vi "Instrument Manager Loop.vi"(8 "System Control":refnum<queue>, 11 "Instrument Manager":refnum<queue>) -> (0 "error out":errorcluster)   [LabVIEW 2020, in "Mock Temperature Controller.lvlib" / "Instrument Manager.lvlib"]
uses:
  Instrument Manager/Instrument Manager.lvlib
  support/Message Queue/Message Cluster.ctl
  Instrument Manager/Instrument State.ctl
  <vilib>/Utility/error.llb/Error Cluster From Error Code.vi
  <vilib>/ErrorRing/Error Ring.xnode
  support/Message Queue/Message Queue.lvlib
  Mock Temperature Controller.lvlib
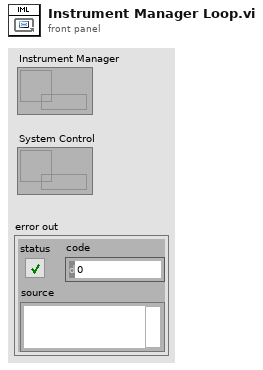
[diagram p1: front panel]
types:
  T1 = typedef "Mock Temperature Controller.lvlib/Instrument Manager.lvlib/Instrument State.ctl" = cluster{"VISA Resource":refnum<visa-resource-name>, "Setpoint":dbl, "Running":bool, "Running Since":timestamp, "Data Point":cluster{"Time Stamp":timestamp, "Value":dbl}, "Current Temperature":dbl, "Sampling Rate (sec/sample)":dbl}
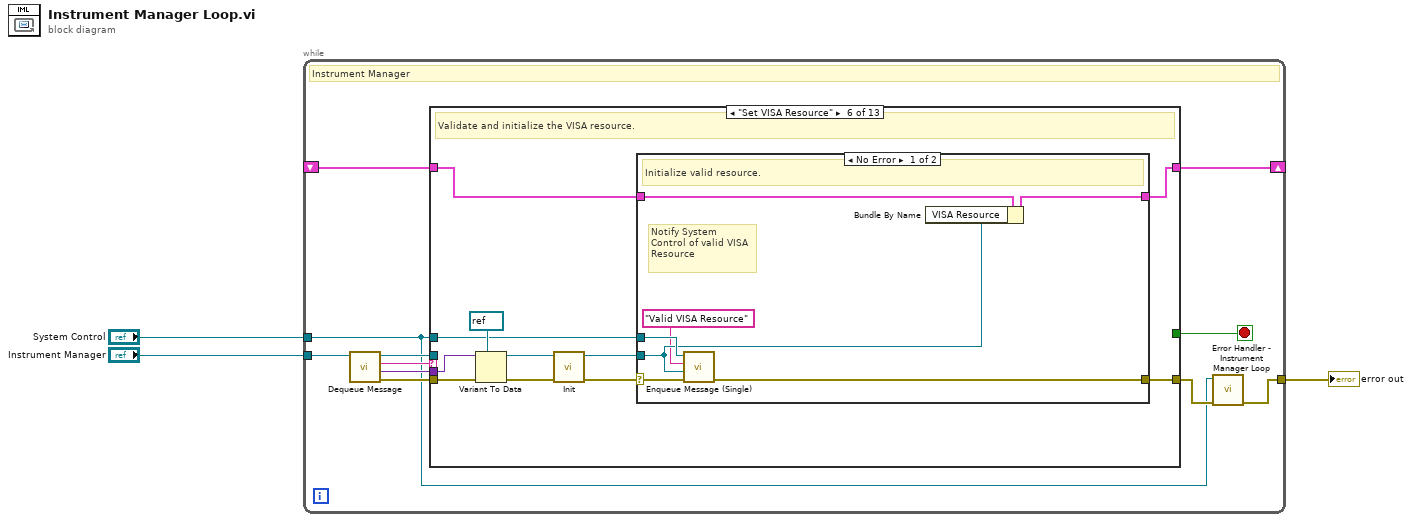
[diagram p0: block diagram]
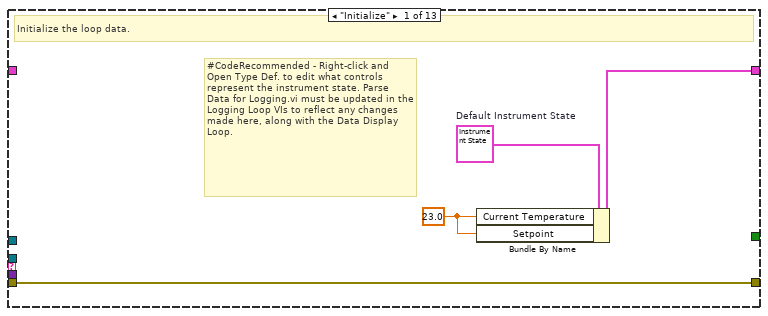
[diagram p2: hidden frame]
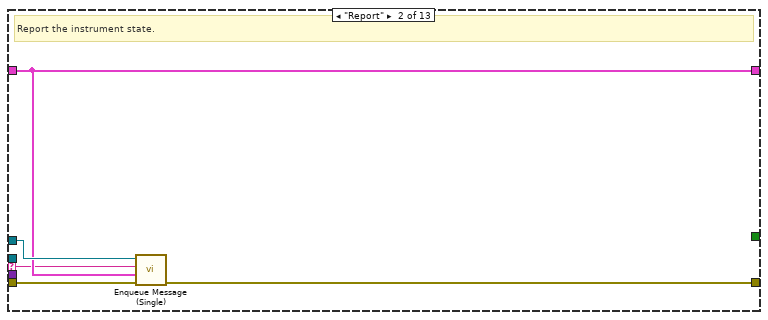
[diagram p3: hidden frame]
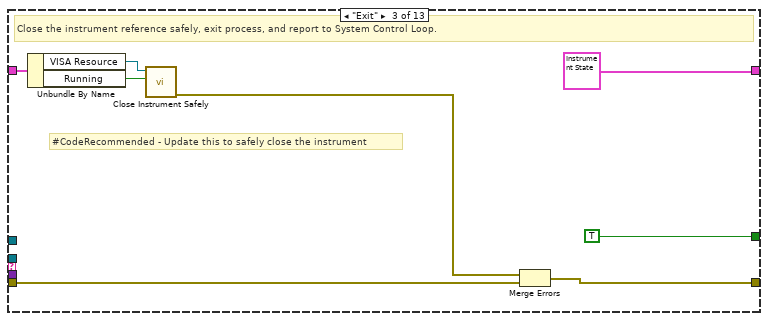
[diagram p4: hidden frame]
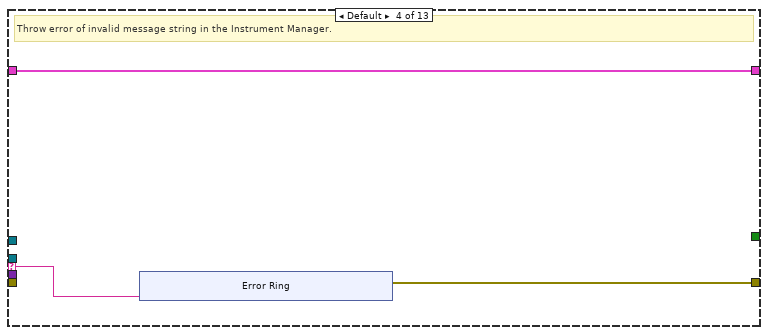
[diagram p5: hidden frame]
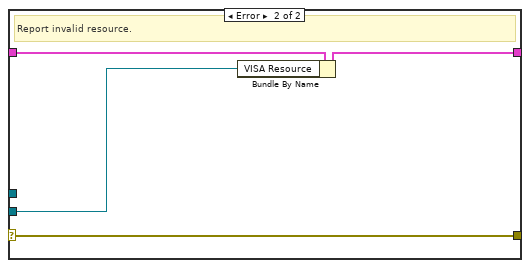
[diagram p7: hidden frame]
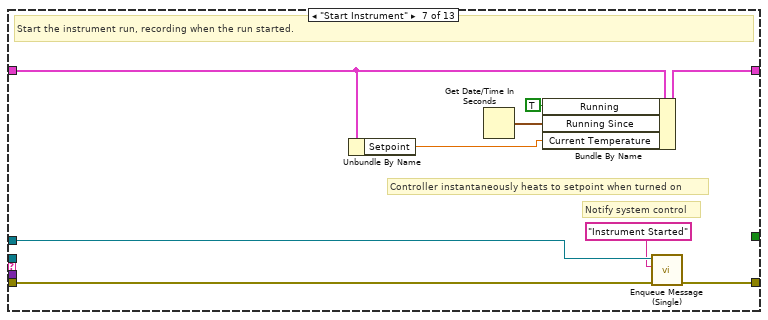
[diagram p8: hidden frame]
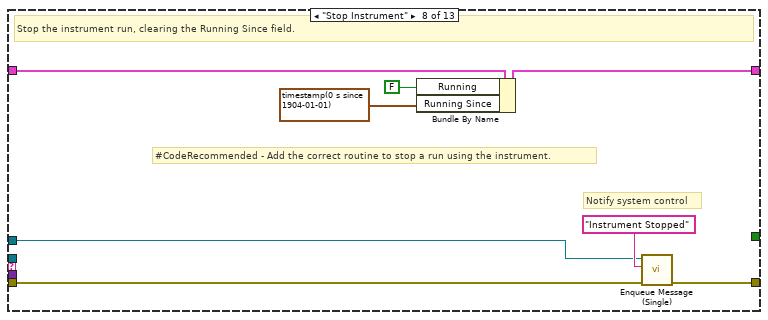
[diagram p9: hidden frame]
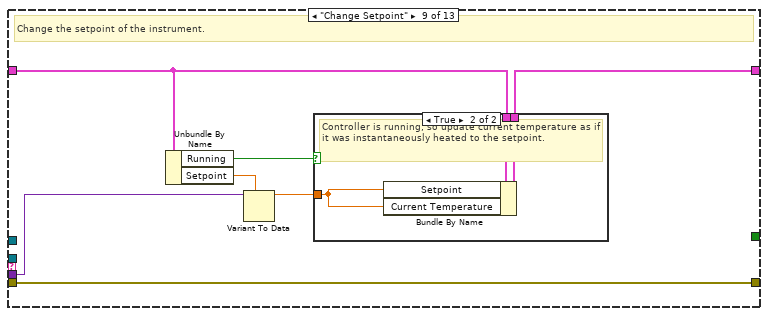
[diagram p10: hidden frame]
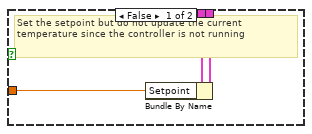
[diagram p11: hidden frame]
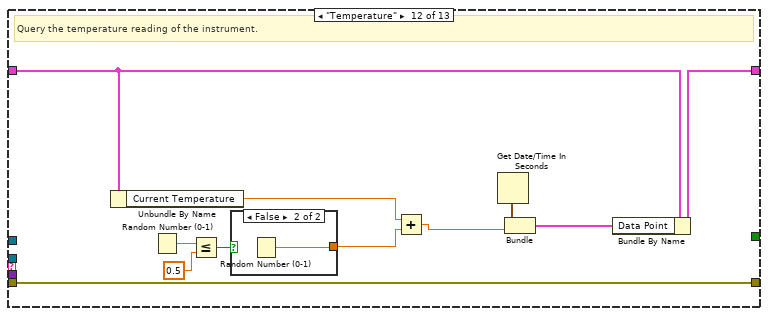
[diagram p14: hidden frame]
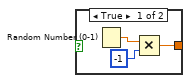
[diagram p15: hidden frame]
diagram:
  n1 = while {
    tunnel: "Instrument Manager" -> [w14]
    tunnel: "System Control" -> [w5]
    tunnel: [w8] -> w1
    shift-right: [w7] -> _
    shift-left: _ -> [w4]
    stop <- w6 stop-if-true
    # "Instrument Manager"
    n2 = call "Dequeue Message.vi"("Message Queue"=w14) -> ("error out"=w10:errorcluster, "Message Data"=w11:variant, "Message"=w13:string, "dup Message Queue"=w12:refnum<queue>)  [unwired: 7 in]
    n3 = case shown="\"Set VISA Resource\"" w13 {
      selector: w13 -> [_ w19 _ w33 _ _ _ _ _ _ _ _ _]
      tunnel: w12 -> [_ _ _ _ _ _ _ _ _ _ _ _ _]
      tunnel: w5 -> [_ w22 _ _ _ w44 w73 w80 _ _ _ _ _]
      tunnel: w11 -> [_ _ _ _ _ w51 _ _ w88 _ _ _ _]
      tunnel: w10 -> [w17 w23 w26 _ w42 w50 w68 w76 w85 w97 w99 w107 w116]
      tunnel: [w17 w21 w25 w32 w42 w54 w74 w82 w85 w97 w99 w107 w116] -> w9
      tunnel: w4 -> [_ w20 w31 w34 w43 w53 w67 w75 w87 w96 w98 w106 w115]
      tunnel: [w16 w20 T1 {"VISA Resource"="", "Setpoint"=0.0, "Running"=FALSE, "Running Since"=timestamp(0 s since 1904-01-01), "Data Point"={"Time Stamp"=timestamp(0 s since 1904-01-01), "Value"=0.0}, "Current Temperature"=0.0, "Sampling Rate (sec/sample)"=0.0} w34 w43 w52 w71 w79 w89 w96 w98 w110 w115] -> w7
      tunnel: [_ _ TRUE _ _ _ _ _ _ _ _ _ _] -> w6
      frame "Initialize" {
        w15 = 23.0 ("Current Temperature")
        w18 = T1 {"VISA Resource"="", "Setpoint"=0.0, "Running"=FALSE, "Running Since"=timestamp(0 s since 1904-01-01), "Data Point"={"Time Stamp"=timestamp(0 s since 1904-01-01), "Value"=0.0}, "Current Temperature"=0.0, "Sampling Rate (sec/sample)"=0.0}  # Default Instrument State
        # "#CodeRecommended - Right-click and Open Type Def. to edit what controls represent the instrument state. Parse Data for Logging.vi must be updated in the Logging Loop VIs to reflect any changes made here, along with the Data Display Loop."
        # "Initialize the loop data."
        n4 = Bundle By Name(cluster=w18, "Current Temperature"=w15, "Setpoint"=w15) -> (w16:T1)
      }
      frame "Report" {
        # "Report the instrument state."
        n5 = call "Enqueue Message (Single).vi"("error in (no error)"=w23, "Message Data"=w20, "Message"=w19, "Message Queue"=w22) -> ("error out"=w21:errorcluster)  [unwired: 6 in, 1 out]
      }
      frame "Exit" {
        # "#CodeRecommended - Update this to safely close the instrument"
        # "Close the instrument reference safely, exit process, and report to System Control Loop."
        n6 = Unbundle By Name(w31) -> ("VISA Resource"=w29:refnum<visa-resource-name>, "Running"=w30:bool)
        n7 = call "Close Instrument Safely.vi"("Running (F)"=w30, "VISA Refnum in"=w29) -> ("error out"=w24:errorcluster)  [unwired: 9 in]
        n8 = Merge Errors(w24, w26) -> (w25:errorcluster)
      }
      frame Default {
        # "Throw error of invalid message string in the Instrument Manager."
        n9 = xnode "Error Ring"("parameter 0"=w33) -> ("error out"=w32:errorcluster)
      }
      frame "--- Copy This Frame ---" {
        # "Copy this frame and add responses to instrument specific messages."
      }
      frame "Set VISA Resource" {
        # "Validate and initialize the VISA resource."
        n10 = Variant To Data(error in=w50, type=refnum<visa-resource-name> refnum, Variant=w51) -> (data=w48:refnum<visa-resource-name>, error out=w49:errorcluster)
        n11 = call "Init.vi"("error in (no error)"=w49, "VISA resource name"=w48) -> ("error out"=w45:errorcluster, "VISA resource out"=w46:refnum<visa-resource-name>)  [unwired: 8 in]
        n12 = case shown="No Error" w45 {
          selector: w45 -> [w60 w62]
          tunnel: w46 -> [w57 w63]
          tunnel: [w59 w62] -> w54
          tunnel: w53 -> [w61 w65]
          tunnel: [w55 w64] -> w52
          tunnel: w44 -> [w58 _]
          frame No Error {
            # "Notify System Control of valid VISA Resource"
            # "Initialize valid resource."
            n13 = call "Enqueue Message (Single).vi"("error in (no error)"=w60, "Message Data"=w57, "Message"="Valid VISA Resource", "Message Queue"=w58) -> ("error out"=w59:errorcluster)  [unwired: 6 in, 1 out]
            n14 = Bundle By Name(cluster=w61, "VISA Resource"=w57) -> (w55:T1)
          }
          frame Error {
            # "Report invalid resource."
            n15 = Bundle By Name(cluster=w65, "VISA Resource"=w63) -> (w64:T1)
          }
        }
      }
      frame "Start Instrument" {
        # "Controller instantaneously heats to setpoint when turned on"
        # "Notify system control"
        # "Start the instrument run, recording when the run started."
        n16 = Unbundle By Name(w67) -> ("Setpoint"=w66:dbl)
        n17 = Get Date/Time In Seconds() -> (seconds since 1Jan1904=w69:timestamp)
        n18 = Bundle By Name(cluster=w67, "Running"=TRUE, "Running Since"=w69, "Current Temperature"=w66) -> (w71:T1)
        n19 = call "Enqueue Message (Single).vi"("error in (no error)"=w68, "Message"="Instrument Started", "Message Queue"=w73) -> ("error out"=w74:errorcluster)  [unwired: 7 in, 1 out]
      }
      frame "Stop Instrument" {
        # "Notify system control"
        # "#CodeRecommended - Add the correct routine to stop a run using the instrument."
        # "Stop the instrument run, clearing the Running Since field."
        n20 = Bundle By Name(cluster=w75, "Running"=FALSE, "Running Since"=timestamp(0 s since 1904-01-01)) -> (w79:T1)
        n21 = call "Enqueue Message (Single).vi"("error in (no error)"=w76, "Message"="Instrument Stopped", "Message Queue"=w80) -> ("error out"=w82:errorcluster)  [unwired: 7 in, 1 out]
      }
      frame "Change Setpoint" {
        # "Change the setpoint of the instrument."
        n22 = Unbundle By Name(w87) -> ("Running"=w83:bool, "Setpoint"=w86:dbl)
        n23 = Variant To Data(type=w86, Variant=w88) -> (data=w84:dbl)  [unwired: 1 in, 1 out]
        n24 = case shown="True" w83 {
          tunnel: [w92 w94] -> w89
          tunnel: w87 -> [w91 w95]
          tunnel: w84 -> [w90 w93]
          frame False {
            # "Set the setpoint but do not update the current temperature since the controller is not running"
            n25 = Bundle By Name(cluster=w91, "Setpoint"=w90) -> (w92:T1)
          }
          frame True {
            # "Controller is running, so update current temperature as if it was instantaneously heated to the setpoint."
            n26 = Bundle By Name(cluster=w95, "Setpoint"=w93, "Current Temperature"=w93) -> (w94:T1)
          }
        }
      }
      frame "--- Copy for Get State Messages ---" {
        # "#CodeNeeded - Use the Bundle by Name function to bundle the new state value into the Instrument State cluster."
        # "#CodeNeeded - Add instrument driver call to query the instrument state requested"
        # "Duplicate this case for messages cases that will query the instrument state."
      }
      frame "Run State" {
        # "In a mock system this doesn't have to do anything"
        # "Query the run state of the instrument."
      }
      frame "Temperature" {
        # "Query the temperature reading of the instrument."
        n27 = Unbundle By Name(w106) -> ("Current Temperature"=w101:dbl)
        n28 = Random Number (0-1)() -> (number: 0 to 1=w105:dbl)
        n29 = Less Or Equal?(x=w105, y=0.5) -> (x <= y?=w103:bool)
        n30 = case shown="False" w103 {
          tunnel: [w111 w114] -> w102
          frame True {
            n31 = Random Number (0-1)() -> (number: 0 to 1=w112:dbl)
            n32 = Multiply(x=w112, y=-1) -> (x*y=w111:dbl)
          }
          frame False {
            n33 = Random Number (0-1)() -> (number: 0 to 1=w114:dbl)
          }
        }
        n34 = Add(x=w101, y=w102) -> (x+y=w100:dbl)
        n35 = Get Date/Time In Seconds() -> (seconds since 1Jan1904=w109:timestamp)
        n36 = Bundle("seconds since 1Jan1904"=w109, w100) -> (w108:cluster{"seconds since 1Jan1904":timestamp, dbl})  [unwired: 1 in]
        n37 = Bundle By Name(cluster=w106, "Data Point"=w108) -> (w110:T1)
      }
      frame "Setpoint" {
        # "Does not need to be checked in a mock system"
        # "Query the setpoint of the instrument."
      }
    }
    n38 = call "Error Handler - Instrument Manager Loop.vi"("error in (no error)"=w9, "Message Queue"=w5) -> ("dup error in"=w8:errorcluster)  [unwired: 8 in, 1 out]
  }
  "error out" <- w1
